vi "Calibrate Mapping.vi"(11 "Image":bool[][](array[boolean])) -> (3 "Image - Mapped":bool[][](array[boolean]))   [LabVIEW 2015]
uses:
  <vilib>/Utility/inputDevices.llb/keyboardAcquire.vi
panel:
  out "keys pressed":T1(array[ring])
  in  "stop":bool
  in  "Keyboard In":refnum<k1>
  out "Keyboard Out":refnum<k1>
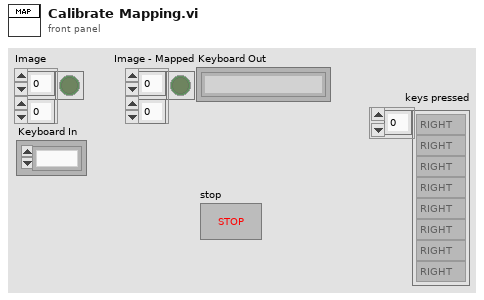
[diagram p1: front panel]
types:
  T1 = enum16{"0", "1", "2", "3", "4", "5", "6", "7", "8", "9", "A", "B", "C", "D", "E", "F", "G", "H", "I", "J", "K", "L", "M", "N", "O", "P", "Q", "R", "S", "T", "U", "V", "W", "X", "Y", "Z", "F1", "F2", "F3", "F4", "F5", "F6", "F7", "F8", "F9", "F10", "F11", "F12", "F13", "F14", "F15", "ADD", "BACK", "BACKSLASH", "CAPITAL", "COMMA", "DECIMAL", "DELETE", "DIVIDE", "DOWN", "END", "EQUALS", "ESCAPE", "GRAVE (`)", "HOME", "INSERT", "LBRACKET", "LCONTROL", "LEFT", "L ALT", "LSHIFT", "LWIN", "MINUS", "MULTIPLY", "NEXT", "NUMLOCK", "NUMPAD_0", "NUMPAD_1", "NUMPAD_2", "NUMPAD_3", "NUMPAD_4", "NUMPAD_5", "NUMPAD_6", "NUMPAD_7", "NUMPAD_8", "NUMPAD_9", "PAUSE", "PERIOD", "PRIOR (PG UP)", "RBRACKET", "RCONTROL", "RETURN", "RIGHT", "R ALT", "RSHIFT", "RWIN", "SCROLL", "SEMICOLON", "SLASH", "SPACE", "SUBTRACT", "TAB", "UP", "ENTER (num pad)", "' (quote)"}[]
  T2 = enum16{"0", "1", "2", "3", "4", "5", "6", "7", "8", "9", "A", "B", "C", "D", "E", "F", "G", "H", "I", "J", "K", "L", "M", "N", "O", "P", "Q", "R", "S", "T", "U", "V", "W", "X", "Y", "Z", "F1", "F2", "F3", "F4", "F5", "F6", "F7", "F8", "F9", "F10", "F11", "F12", "F13", "F14", "F15", "ADD", "BACK", "BACKSLASH", "CAPITAL", "COMMA", "DECIMAL", "DELETE", "DIVIDE", "DOWN", "END", "EQUALS", "ESCAPE", "GRAVE (`)", "HOME", "INSERT", "LBRACKET", "LCONTROL", "LEFT", "L ALT", "LSHIFT", "LWIN", "MINUS", "MULTIPLY", "NEXT", "NUMLOCK", "NUMPAD_0", "NUMPAD_1", "NUMPAD_2", "NUMPAD_3", "NUMPAD_4", "NUMPAD_5", "NUMPAD_6", "NUMPAD_7", "NUMPAD_8", "NUMPAD_9", "PAUSE", "PERIOD", "PRIOR (PG UP)", "RBRACKET", "RCONTROL", "RETURN", "RIGHT", "R ALT", "RSHIFT", "RWIN", "SCROLL", "SEMICOLON", "SLASH", "SPACE", "SUBTRACT", "TAB", "UP", "ENTER (num pad)", "' (quote)"}
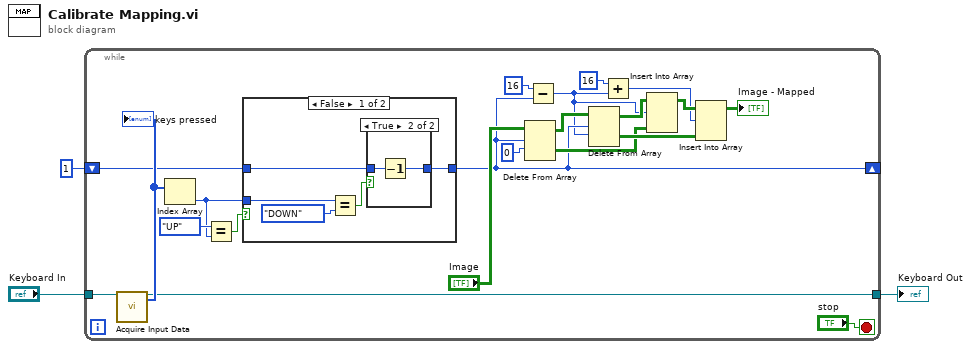
[diagram p0: block diagram]
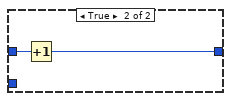
[diagram p3: hidden frame]
diagram:
  n1 = while {
    shift-right: [w10] -> _
    shift-left: 1 -> [w12]
    tunnel: "Keyboard In" -> [w5]
    tunnel: [w4] -> w2
    stop <- "stop" stop-if-true
    n2 = call-poly <vilib>:"Acquire Input Data.vi"("device ID"=w5) -> ("device ID"=w4:refnum<k1>, "keys pressed"=w15:T1)  [unwired: 16 in, 1 out]
    "keys pressed" <- w15
    n3 = Index Array(array=w15) -> (element=w11:T2)  [unwired: 1 in]
    n4 = Equal?(x=T2."UP" ("y"), y=w11) -> (x = y?=w13:bool)
    n5 = case shown="False" w13 {
      tunnel: w12 -> [w26 w33]
      tunnel: [w25 w34] -> w10
      tunnel: w11 -> [w29 _]
      frame False {
        n6 = Equal?(x=w29, y=T2."DOWN") -> (x = y?=w27:bool)
        n7 = case shown="True" w27 {
          tunnel: w26 -> [w30 w31]
          tunnel: [w30 w32] -> w25
          frame False {
          }
          frame True {
            n8 = Decrement(x=w31) -> (x-1=w32:i32)
          }
        }
      }
      frame True {
        n9 = Increment(x=w33) -> (x+1=w34:i32)
      }
    }
    n10 = Delete From Array(array="Image", length=w10, index (row)=0) -> (deleted portion=w22:bool[][], array with subset deleted=w21:bool[][])  [unwired: 1 in]
    n11 = Subtract(x=16, y=w10) -> (x-y=w8:i32)
    n12 = Delete From Array(array=w21, length=w10, index (row)=w8) -> (deleted portion=w24:bool[][], array with subset deleted=w18:bool[][])  [unwired: 1 in]
    n13 = Add(x=16, y=w8) -> (x+y=w6:i32)
    n14 = Insert Into Array(array=w18, index (row)=w8, new element=w22) -> (w23:bool[][])  [unwired: 1 in]
    n15 = Insert Into Array(array=w23, index (row)=w6, new element=w24) -> (→"Image - Mapped":bool[][])  [unwired: 1 in]
  }
  "Keyboard Out" <- w2
